vi "Main.vi"() -> ()   [LabVIEW 2018] (continued)
              }
              frame Enabled {
              }
            }
            n1833 = disable-structure shown="启用" {
              disable-tunnel: [w775 w777] -> w747
              disable-tunnel: w743 -> [w774 w777]
              frame Disabled {
                n1834 = call <vilib>:"Boolean Crossing PtByPt.vi"("direction"=enum16{"either", "false-true", "true-false"}."true-false", "input"=w774) -> ("crossing"=w775:bool)  [unwired: 1 in]
              }
              frame Enabled {
              }
            }
            n1835 = call <vilib>:"Boolean Crossing PtByPt.vi"("direction"=enum16{"either", "false-true", "true-false"}."false-true", "input"=w746) -> ("crossing"=w752:bool)  [unwired: 1 in]
            n1836 = case shown="真" w752 {
              tunnel: w754 -> [w815 w820]
              tunnel: w753 -> [w814 w821]
              tunnel: [w815 w819] -> w751
              tunnel: [w814 w818] -> w750
              frame False {
              }
              frame True {
                w829 = u16 0 items=["byte", "word", "Dword"] ("数据类型")
                w827 = u8 132 items=["I/O (P)"=128, "Input (I)"=129, "Output (Q)"=130, "Bit Memory (M)"=131, "Data (DB)"=132, "Instance Data (DI)"=133, "Local Data (L)"=134, "Predecessor Local Data (VL)"=135] ("寄存器类型")
                n1837 = call "S7_Read.vi"("TCP"=w820, "DB #"=u16 20, "读取长度"=u16 13, "寄存器类型"=w827, "起始地址"=u32 6, "数据类型"=w829, "error in"=w821) -> ("TCP"=w819:refnum<k5>, "数据"=w824:u32[], "error out"=w822:errorcluster)  [unwired: 5 in, 1 out]
                n1838 = To Unsigned Word Integer(number=w824) -> (unsigned 16bit integer=w823:u16[])
                n1839 = call "还原为字符串.vi"("error in (no error)"=w822, "输入数组"=w823) -> ("error out"=w817:errorcluster, "字符串"=w816:string)  [unwired: 8 in]
                n1840 = stacked-sequence {
                  tunnel: [_ w833] -> w818
                  tunnel: w817 -> [_ w832]
                  tunnel: w816 -> [w830 _]
                  frame #0 {
                    "80二维码" <- w830
                  }
                  frame #1 {
                    n1841 = property on="ST80扫码请求 （事件）" class="Bool (严格)"(error in=w832, "Val(Sgnl)"=TRUE ("值(信号)")) -> (error out=w833:errorcluster)  [unwired: 1 in, 1 out]
                  }
                }
              }
            }
            n1842 = case shown="假" w744 {
              frame False {
                n1843 = local write "80扫码回复写入"(FALSE ("201扫码回复写入")) -> ()
              }
              frame True {
              }
            }
            n1844 = case shown="假" w747 {
              frame False {
                n1845 = local write "80数据回复写入"(FALSE ("201数据回复写入")) -> ()
              }
              frame True {
              }
            }
            n1846 = call <vilib>:"Boolean Crossing PtByPt.vi"("direction"=enum16{"either", "false-true", "true-false"}."false-true", "input"=w743) -> ("crossing"=w748:bool)  [unwired: 1 in]
            n1847 = case shown="真" w748 {
              tunnel: [w781 w788] -> w742
              tunnel: [w780 w783] -> w741
              tunnel: w750 -> [w780 w789]
              tunnel: w751 -> [w781 w790]
              frame False {
              }
              frame True {
                w794 = u16 1 items=["byte", "word", "Dword"] ("数据类型")
                w796 = u8 132 items=["I/O (P)"=128, "Input (I)"=129, "Output (Q)"=130, "Bit Memory (M)"=131, "Data (DB)"=132, "Instance Data (DI)"=133, "Local Data (L)"=134, "Predecessor Local Data (VL)"=135] ("寄存器类型")
                n1848 = call "S7_Read.vi"("TCP"=w790, "DB #"=u16 20, "读取长度"=u16 1, "寄存器类型"=w796, "起始地址"=u32 20, "数据类型"=w794, "error in"=w789) -> ("TCP"=w788:refnum<k5>, "数据"=w802:u32[], "error out"=w784:errorcluster)  [unwired: 5 in, 1 out]
                n1849 = local read "ST80_Spring_plate_5025473"() -> (w785:string)
                n1850 = local read "ST80_Flat_sael_5020064"() -> (w787:string)
                n1851 = local read "ST80_Spring_5024883"() -> (w786:string)
                n1852 = Index Array(array=w802) -> (element=w804:u32)  [unwired: 1 in]
                n1853 = Equal?(x=w804, y=u32 1) -> (x = y?=w803:bool)
                n1854 = case shown="真" w803 {
                  tunnel: ["NG" "OK"] -> w807
                  frame False {
                  }
                  frame True {
                  }
                }
                n1855 = Format Date/Time String(time format string (%c)="%Y-%m-%d" ("时间格式字符串(%c)")) -> (date/time string=w805:string)  [unwired: 2 in]
                n1856 = Get Date/Time String(want seconds? (F)=TRUE ("需要秒？(F)")) -> (time string=w806:string)  [unwired: 2 in, 1 out]
                n1857 = Insert Into Array(array=string[] [] ("数组"), index=0 ("索引"), new element #1="80" ("新元素/子数组"), new element #2=w807, new element #3=w805, new element #4=w806, new element #5=w807, new element #6=w787, new element #7=w786, new element #8=w785) -> (w782:string[])
                n1858 = stacked-sequence {
                  tunnel: w784 -> [_ w811]
                  tunnel: [_ w810] -> w783
                  tunnel: w782 -> [w808 _]
                  frame #0 {
                    "80数据" <- w808
                  }
                  frame #1 {
                    n1859 = property on="ST80数据保存请求（事件）" class="Bool (严格)"(error in=w811, "Val(Sgnl)"=TRUE ("值(信号)")) -> (error out=w810:errorcluster)  [unwired: 1 in, 1 out]
                  }
                }
              }
            }
          }
          frame "写" {
            w843 = u8 132 items=["I/O (P)"=128, "Input (I)"=129, "Output (Q)"=130, "Bit Memory (M)"=131, "Data (DB)"=132, "Instance Data (DI)"=133, "Local Data (L)"=134, "Predecessor Local Data (VL)"=135] ("寄存器类型")
            w842 = u16 1 items=["byte", "word", "Dword"] ("数据类型")
            w855 = u8 132 items=["I/O (P)"=128, "Input (I)"=129, "Output (Q)"=130, "Bit Memory (M)"=131, "Data (DB)"=132, "Instance Data (DI)"=133, "Local Data (L)"=134, "Predecessor Local Data (VL)"=135] ("寄存器类型")
            w854 = u16 1 items=["byte", "word", "Dword"] ("数据类型")
            w862 = u8 132 items=["I/O (P)"=128, "Input (I)"=129, "Output (Q)"=130, "Bit Memory (M)"=131, "Data (DB)"=132, "Instance Data (DI)"=133, "Local Data (L)"=134, "Predecessor Local Data (VL)"=135] ("寄存器类型")
            w859 = u16 1 items=["byte", "word", "Dword"] ("数据类型")
            n1860 = local read "80看门狗"() -> (w853:i32)
            n1861 = case shown="0" w853 {
              tunnel: [0 ("y") 1 ("y")] -> w852
              frame 1, Default {
              }
              frame 0 {
              }
            }
            "80看门狗" <- w852
            n1862 = call "S7_Write.vi"("TCP"=w858, "寄存器类型"=w862, "DB #"=u16 20, "写入地址"=u32 54, "数据类型"=w859, "写入数据"=w852) -> ("TCP"=w851:refnum<k5>, "error out"=w850:errorcluster)  [unwired: 7 in, 1 out]
            n1863 = case shown="真" "80扫码回复写入" {
              tunnel: w851 -> [w881 w889]
              tunnel: w850 -> [w880 w888]
              tunnel: [w881 w887] -> w848
              tunnel: [w880 w886] -> w847
              tunnel: [999 w885] -> w846
              frame False {
              }
              frame True {
                w897 = u8 132 items=["I/O (P)"=128, "Input (I)"=129, "Output (Q)"=130, "Bit Memory (M)"=131, "Data (DB)"=132, "Instance Data (DI)"=133, "Local Data (L)"=134, "Predecessor Local Data (VL)"=135] ("寄存器类型")
                w896 = u16 1 items=["byte", "word", "Dword"] ("数据类型")
                w891 = u8 132 items=["I/O (P)"=128, "Input (I)"=129, "Output (Q)"=130, "Bit Memory (M)"=131, "Data (DB)"=132, "Instance Data (DI)"=133, "Local Data (L)"=134, "Predecessor Local Data (VL)"=135] ("寄存器类型")
                w892 = u16 1 items=["byte", "word", "Dword"] ("数据类型")
                n1864 = local read "上一站号 (80)"() -> (w884:string)
                n1865 = local read "上一站结果 (80)"() -> (w883:string)
                n1866 = Decimal String To Number(string=w884, default (0L)=u32 0 ("默认(0 I32)")) -> (number=w901:u32)  [unwired: 1 in, 1 out]
                n1867 = call "S7_Write.vi"("TCP"=w889, "寄存器类型"=w891, "DB #"=u16 20, "写入地址"=u32 28, "数据类型"=w892, "写入数据"=w901, "error in"=w888) -> ("TCP"=w900:refnum<k5>, "error out"=w899:errorcluster)  [unwired: 6 in, 1 out]
                n1868 = Equal?(x=w883, y="OK") -> (x = y?=w903:bool)
                n1869 = case shown="假" w903 {
                  tunnel: [u32 2 ("写入数据") u32 1 ("写入数据")] -> w904
                  frame False {
                  }
                  frame True {
                  }
                }
                n1870 = local read "扫码请求回复80"() -> (w882:string)
                n1871 = call "S7_Write.vi"("TCP"=w900, "寄存器类型"=w897, "DB #"=u16 20, "写入地址"=u32 30, "数据类型"=w896, "写入数据"=w904, "error in"=w899) -> ("TCP"=w887:refnum<k5>, "error out"=w886:errorcluster)  [unwired: 6 in, 1 out]
                n1872 = Decimal String To Number(string=w882) -> (number=w885:i32)  [unwired: 2 in, 1 out]
              }
            }
            n1873 = call "S7_Write.vi"("TCP"=w848, "寄存器类型"=w855, "DB #"=u16 20, "写入地址"=u32 2, "数据类型"=w854, "写入数据"=w846, "error in"=w847) -> ("TCP"=w841:refnum<k5>, "error out"=w840:errorcluster)  [unwired: 6 in, 1 out]
            n1874 = case shown="真" "80数据回复写入" {
              tunnel: [999 w878] -> w839
              frame False {
              }
              frame True {
                n1875 = local read "数据保存请求回复80"() -> (w877:string)
                n1876 = Decimal String To Number(string=w877) -> (number=w878:i32)  [unwired: 2 in, 1 out]
              }
            }
            n1877 = call "S7_Write.vi"("TCP"=w841, "寄存器类型"=w843, "DB #"=u16 20, "写入地址"=u32 4, "数据类型"=w842, "写入数据"=w839, "error in"=w840) -> ("TCP"=w837:refnum<k5>, "error out"=w835:errorcluster)  [unwired: 6 in, 1 out]
            n1878 = disable-structure shown="启用" {
              disable-tunnel: w837 -> [w865 w869]
              disable-tunnel: [w865 w872] -> w836
              disable-tunnel: w835 -> [w866 w870]
              disable-tunnel: [w866 w871] -> w834
              frame Disabled {
              }
              frame Enabled {
                w874 = u8 132 items=["I/O (P)"=128, "Input (I)"=129, "Output (Q)"=130, "Bit Memory (M)"=131, "Data (DB)"=132, "Instance Data (DI)"=133, "Local Data (L)"=134, "Predecessor Local Data (VL)"=135] ("寄存器类型")
                w868 = u16 1 items=["byte", "word", "Dword"] ("数据类型")
                n1879 = local read "产品型号"() -> (w867:u32)
                n1880 = call "S7_Write.vi"("TCP"=w869, "寄存器类型"=w874, "DB #"=u16 20, "写入地址"=u32 56, "数据类型"=w868, "写入数据"=w867, "error in"=w870) -> ("TCP"=w872:refnum<k5>, "error out"=w871:errorcluster)  [unwired: 6 in, 1 out]
              }
            }
          }
          frame "错误" {
            n1881 = call "S7_Close.vi"("TCP Connection Ref"=w911) -> ("error out"=w912:errorcluster)  [unwired: 10 in]
            n1882 = call <vilib>:"Clear Errors.vi"("error in (no error)"=w912) -> ()  [unwired: 5 in, 2 out]
          }
          frame "退出" {
            n1883 = call "S7_Close.vi"("TCP Connection Ref"=w918) -> ("error out"=w919:errorcluster)  [unwired: 10 in]
            n1884 = call <vilib>:"Clear Errors.vi"("error in (no error)"=w919) -> ()  [unwired: 5 in, 2 out]
          }
        }
      }
      n1885 = while {
        shift-right: [w2621] -> _
        shift-left: errorcluster {"status"=FALSE, "code"=0, "source"=""} ("错误常量") -> [w2624]
        shift-right: [w2620] -> _
        shift-left: enum16{"初始化", "读", "写", "错误", "退出"}."初始化" -> [w2625]
        shift-right: [w2622] -> _
        shift-left: _ -> [w2619]
        stop <- w2618 stop-if-true
        n1886 = local read "退出"() -> (w2626:bool)
        n1887 = case shown="假" w2626 {
          tunnel: w2625 -> [w2627 _]
          tunnel: [w2628 enum16{"初始化", "读", "写", "错误", "退出"}."退出"] -> w2617
          tunnel: w2624 -> [w2629 _]
          frame False {
            n1888 = case shown="错误" w2629 {
              tunnel: [w2630 enum16{"初始化", "读", "写", "错误", "退出"}."错误"] -> w2628
              tunnel: w2627 -> [w2630 _]
              frame No Error {
              }
              frame Error {
              }
            }
          }
          frame True {
          }
        }
        n1889 = Wait (ms)(milliseconds to wait=u32 80 ("等待时间（毫秒）")) -> ()  [unwired: 1 out]
        n1890 = case shown="\"写\"" w2617 {
          tunnel: [w2635 w2676 w2846 refnum<k5> refnum ("TCP") refnum<k5> refnum ("TCP")] -> w2622
          tunnel: [w2633 w2677 w2844 errorcluster {"status"=FALSE, "code"=0, "source"=""} ("error out") errorcluster {"status"=FALSE, "code"=0, "source"=""} ("error out")] -> w2621
          tunnel: [enum16{"初始化", "读", "写", "错误", "退出"}."读" enum16{"初始化", "读", "写", "错误", "退出"}."写" enum16{"初始化", "读", "写", "错误", "退出"}."读" enum16{"初始化", "读", "写", "错误", "退出"}."初始化" enum16{"初始化", "读", "写", "错误", "退出"}."退出"] -> w2620
          tunnel: w2619 -> [_ w2696 w2886 w2969 w2976]
          tunnel: [FALSE FALSE FALSE FALSE TRUE] -> w2618
          frame "初始化", Default {
            w2648 = u16 0 items=["byte", "word", "Dword"] ("数据类型")
            w2646 = u8 132 items=["I/O (P)"=128, "Input (I)"=129, "Output (Q)"=130, "Bit Memory (M)"=131, "Data (DB)"=132, "Instance Data (DI)"=133, "Local Data (L)"=134, "Predecessor Local Data (VL)"=135] ("寄存器类型")
            w2649 = u16 0 items=["byte", "word", "Dword"] ("数据类型")
            w2651 = u8 132 items=["I/O (P)"=128, "Input (I)"=129, "Output (Q)"=130, "Bit Memory (M)"=131, "Data (DB)"=132, "Instance Data (DI)"=133, "Local Data (L)"=134, "Predecessor Local Data (VL)"=135] ("寄存器类型")
            w2661 = u8 0 items=["S7-1200.200.200SMART"=0, "S7-300"=2, "S7-400"=3] ("PLC 系列")
            n1891 = call "S7_Open.vi"("IP 地址"="192.168.1.40", "PLC 系列"=w2661, "超时（MS）"=100) -> ("TCP"=w2636:refnum<k5>, "error out"=w2634:errorcluster)  [unwired: 10 in, 1 out]
            n1892 = case shown="错误" w2634 {
              tunnel: [FALSE TRUE] -> w2657
              frame No Error {
              }
              frame Error {
              }
            }
            n1893 = local write "ST40通讯状态"(w2657) -> ()
            n1894 = call "S7_Read.vi"("TCP"=w2636, "DB #"=u16 20, "读取长度"=u16 13, "寄存器类型"=w2646, "起始地址"=u32 22, "数据类型"=w2648, "error in"=w2634) -> ("TCP"=w2639:refnum<k5>, "数据"=w2643:u32[], "error out"=w2641:errorcluster)  [unwired: 5 in, 1 out]
            n1895 = To Unsigned Word Integer(number=w2643) -> (unsigned 16bit integer=w2642:u16[])
            n1896 = call "还原为字符串.vi"("error in (no error)"=w2641, "输入数组"=w2642) -> ("error out"=w2638:errorcluster, "字符串"=w2640:string)  [unwired: 8 in]
            n1897 = local write "401二维码"(w2640) -> ()
            n1898 = call "S7_Read.vi"("TCP"=w2639, "DB #"=u16 20, "读取长度"=u16 13, "寄存器类型"=w2651, "起始地址"=u32 44, "数据类型"=w2649, "error in"=w2638) -> ("TCP"=w2635:refnum<k5>, "数据"=w2654:u32[], "error out"=w2656:errorcluster)  [unwired: 5 in, 1 out]
            n1899 = To Unsigned Word Integer(number=w2654) -> (unsigned 16bit integer=w2655:u16[])
            n1900 = call "还原为字符串.vi"("error in (no error)"=w2656, "输入数组"=w2655) -> ("error out"=w2633:errorcluster, "字符串"=w2637:string)  [unwired: 8 in]
            n1901 = local write "402二维码"(w2637) -> ()
          }
          frame "读" {
            w2697 = u16 0 items=["byte", "word", "Dword"] ("数据类型")
            w2699 = u8 132 items=["I/O (P)"=128, "Input (I)"=129, "Output (Q)"=130, "Bit Memory (M)"=131, "Data (DB)"=132, "Instance Data (DI)"=133, "Local Data (L)"=134, "Predecessor Local Data (VL)"=135] ("寄存器类型")
            n1902 = call "S7_Read.vi"("TCP"=w2696, "DB #"=u16 20, "读取长度"=u16 1, "寄存器类型"=w2699, "起始地址"=u32 0, "数据类型"=w2697) -> ("TCP"=w2694:refnum<k5>, "数据"=w2704:u32[], "读取成功"=w2707:bool, "error out"=w2693:errorcluster)  [unwired: 6 in]
            n1903 = Not(x=w2707) -> (.not. x?=→"ST40通讯状态":bool)
            n1904 = Index Array(array=w2704, index=0 ("索引")) -> (element=w2705:u32)
            n1905 = Number To Boolean Array(number=w2705) -> (Boolean array=w2706:bool[])
            n1906 = Index Array(array=w2706, index #1=0 ("索引"), index #5=6 ("索引")) -> (element #1=w2683:bool, element #2=w2671:bool, element #3=w2669:bool, element #4=w2668:bool, element #5=w2666:bool, element #6=w2665:bool)  [unwired: 4 in]
            "ST401扫码请求" <- w2683
            "ST401数据保存请求" <- w2671
            "ST402扫码请求" <- w2669
            "ST402数据保存请求" <- w2668
            n1907 = call <vilib>:"Boolean Crossing PtByPt.vi"("direction"=enum16{"either", "false-true", "true-false"}."false-true", "input"=w2683) -> ("crossing"=w2692:bool)  [unwired: 1 in]
            n1908 = disable-structure shown="启用" {
              disable-tunnel: [w2712 w2713] -> w2684
              disable-tunnel: w2669 -> [w2710 w2713]
              frame Disabled {
                n1909 = call <vilib>:"Boolean Crossing PtByPt.vi"("direction"=enum16{"either", "false-true", "true-false"}."true-false", "input"=w2710) -> ("crossing"=w2712:bool)  [unwired: 1 in]
              }
              frame Enabled {
              }
            }
            n1910 = disable-structure shown="启用" {
              disable-tunnel: [w2723 w2725] -> w2685
              disable-tunnel: w2671 -> [w2722 w2725]
              frame Disabled {
                n1911 = call <vilib>:"Boolean Crossing PtByPt.vi"("direction"=enum16{"either", "false-true", "true-false"}."true-false", "input"=w2722) -> ("crossing"=w2723:bool)  [unwired: 1 in]
              }
              frame Enabled {
              }
            }
            n1912 = case shown="真" w2692 {
              tunnel: w2694 -> [w2825 w2830]
              tunnel: w2693 -> [w2824 w2831]
              tunnel: [w2825 w2829] -> w2691
              tunnel: [w2824 w2828] -> w2690
              frame False {
              }
              frame True {
                w2839 = u16 0 items=["byte", "word", "Dword"] ("数据类型")
                w2837 = u8 132 items=["I/O (P)"=128, "Input (I)"=129, "Output (Q)"=130, "Bit Memory (M)"=131, "Data (DB)"=132, "Instance Data (DI)"=133, "Local Data (L)"=134, "Predecessor Local Data (VL)"=135] ("寄存器类型")
                n1913 = call "S7_Read.vi"("TCP"=w2830, "DB #"=u16 20, "读取长度"=u16 13, "寄存器类型"=w2837, "起始地址"=u32 22, "数据类型"=w2839, "error in"=w2831) -> ("TCP"=w2829:refnum<k5>, "数据"=w2834:u32[], "error out"=w2832:errorcluster)  [unwired: 5 in, 1 out]
                n1914 = To Unsigned Word Integer(number=w2834) -> (unsigned 16bit integer=w2833:u16[])
                n1915 = call "还原为字符串.vi"("error in (no error)"=w2832, "输入数组"=w2833) -> ("error out"=w2827:errorcluster, "字符串"=w2826:string)  [unwired: 8 in]
                n1916 = stacked-sequence {
                  tunnel: [_ w2843] -> w2828
                  tunnel: w2827 -> [_ w2842]
                  tunnel: w2826 -> [w2840 _]
                  frame #0 {
                    "401二维码" <- w2840
                  }
                  frame #1 {
                    n1917 = property on="ST401扫码请求（事件）" class="Bool (严格)"(error in=w2842, "Val(Sgnl)"=TRUE ("值(信号)")) -> (error out=w2843:errorcluster)  [unwired: 1 in, 1 out]
                  }
                }
              }
            }
            n1918 = disable-structure shown="启用" {
              disable-tunnel: enum16{"either", "false-true", "true-false"}."true-false" ("direction") -> [w2716 _]
              disable-tunnel: w2683 -> [w2715 w2717]
              disable-tunnel: [w2714 w2717] -> w2672
              frame Disabled {
                n1919 = call <vilib>:"Boolean Crossing PtByPt.vi"("direction"=w2716, "input"=w2715) -> ("crossing"=w2714:bool)  [unwired: 1 in]
              }
              frame Enabled {
              }
            }
            n1920 = case shown="假" w2672 {
              frame False {
                n1921 = local write "401扫码回复写入"(FALSE ("201扫码回复写入")) -> ()
              }
              frame True {
              }
            }
            n1922 = case shown="假" w2684 {
              frame False {
                n1923 = local write "402扫码回复写入"(FALSE ("202扫码回复写入")) -> ()
              }
              frame True {
              }
            }
            n1924 = case shown="假" w2685 {
              frame False {
                n1925 = local write "401数据回复写入"(FALSE ("201数据回复写入")) -> ()
              }
              frame True {
              }
            }
            n1926 = disable-structure shown="启用" {
              disable-tunnel: [w2719 w2721] -> w2670
              disable-tunnel: w2668 -> [w2718 w2721]
              frame Disabled {
                n1927 = call <vilib>:"Boolean Crossing PtByPt.vi"("direction"=enum16{"either", "false-true", "true-false"}."true-false", "input"=w2718) -> ("crossing"=w2719:bool)  [unwired: 1 in]
              }
              frame Enabled {
              }
            }
            n1928 = call <vilib>:"Boolean Crossing PtByPt.vi"("direction"=enum16{"either", "false-true", "true-false"}."false-true", "input"=w2671) -> ("crossing"=w2688:bool)  [unwired: 1 in]
            n1929 = case shown="真" w2688 {
              tunnel: [w2788 w2796] -> w2682
              tunnel: [w2787 w2790] -> w2681
              tunnel: w2690 -> [w2787 w2797]
              tunnel: w2691 -> [w2788 w2798]
              tunnel: w2666 -> [_ w2793]
              frame False {
              }
              frame True {
                w2802 = u16 1 items=["byte", "word", "Dword"] ("数据类型")
                w2804 = u8 132 items=["I/O (P)"=128, "Input (I)"=129, "Output (Q)"=130, "Bit Memory (M)"=131, "Data (DB)"=132, "Instance Data (DI)"=133, "Local Data (L)"=134, "Predecessor Local Data (VL)"=135] ("寄存器类型")
                n1930 = case shown="假" w2793 {
                  tunnel: ["F" "T"] -> w2792
                  frame False {
                  }
                  frame True {
                  }
                }
                n1931 = call "S7_Read.vi"("TCP"=w2798, "DB #"=u16 20, "读取长度"=u16 2, "寄存器类型"=w2804, "起始地址"=u32 64, "数据类型"=w2802, "error in"=w2797) -> ("TCP"=w2796:refnum<k5>, "数据"=w2810:u32[], "error out"=w2791:errorcluster)  [unwired: 5 in, 1 out]
                n1932 = Index Array(array=w2810) -> (element #1=w2812:u32, element #2=w2795:u32)  [unwired: 2 in]
                n1933 = Equal?(x=w2812, y=u32 1) -> (x = y?=w2811:bool)
                n1934 = case shown="真" w2811 {
                  tunnel: ["NG" "OK"] -> w2815
                  frame False {
                  }
                  frame True {
                  }
                }
                n1935 = Number To Decimal String(number=w2795) -> (decimal integer string=w2794:string)  [unwired: 1 in]
                n1936 = Format Date/Time String(time format string (%c)="%Y-%m-%d" ("时间格式字符串(%c)")) -> (date/time string=w2813:string)  [unwired: 2 in]
                n1937 = Get Date/Time String(want seconds? (F)=TRUE ("需要秒？(F)")) -> (time string=w2814:string)  [unwired: 2 in, 1 out]
                n1938 = Insert Into Array(array=string[] [] ("数组"), index=0 ("索引"), new element #1="401" ("新元素/子数组"), new element #2=w2815, new element #3=w2813, new element #4=w2814, new element #5=w2815, new element #6=w2794, new element #7=w2792) -> (w2789:string[])
                n1939 = stacked-sequence {
                  tunnel: w2791 -> [_ w2819]
                  tunnel: [_ w2818] -> w2790
                  tunnel: w2789 -> [w2816 _]
                  frame #0 {
                    "401数据" <- w2816
                  }
                  frame #1 {
                    n1940 = property on="ST401数据读取（事件）" class="Bool (严格)"(error in=w2819, "Val(Sgnl)"=TRUE ("值(信号)")) -> (error out=w2818:errorcluster)  [unwired: 1 in, 1 out]
                  }
                }
              }
            }
            n1941 = case shown="假" w2670 {
              frame False {
                n1942 = local write "402数据回复写入"(FALSE ("202数据回复写入")) -> ()
              }
              frame True {
              }
            }
            n1943 = call <vilib>:"Boolean Crossing PtByPt.vi"("direction"=enum16{"either", "false-true", "true-false"}."false-true", "input"=w2669) -> ("crossing"=w2680:bool)  [unwired: 1 in]
            n1944 = case shown="真" w2680 {
              tunnel: w2682 -> [w2765 w2771]
              tunnel: w2681 -> [w2764 w2770]
              tunnel: [w2764 w2767] -> w2678
              tunnel: [w2765 w2769] -> w2679
              frame False {
              }
              frame True {
                w2772 = u16 0 items=["byte", "word", "Dword"] ("数据类型")
                w2774 = u8 132 items=["I/O (P)"=128, "Input (I)"=129, "Output (Q)"=130, "Bit Memory (M)"=131, "Data (DB)"=132, "Instance Data (DI)"=133, "Local Data (L)"=134, "Predecessor Local Data (VL)"=135] ("寄存器类型")
                n1945 = call "S7_Read.vi"("TCP"=w2771, "DB #"=u16 20, "读取长度"=u16 13, "寄存器类型"=w2774, "起始地址"=u32 44, "数据类型"=w2772, "error in"=w2770) -> ("TCP"=w2769:refnum<k5>, "数据"=w2777:u32[], "error out"=w2779:errorcluster)  [unwired: 5 in, 1 out]
                n1946 = To Unsigned Word Integer(number=w2777) -> (unsigned 16bit integer=w2778:u16[])
                n1947 = call "还原为字符串.vi"("error in (no error)"=w2779, "输入数组"=w2778) -> ("error out"=w2768:errorcluster, "字符串"=w2766:string)  [unwired: 8 in]
                n1948 = stacked-sequence {
                  tunnel: w2768 -> [_ w2783]
                  tunnel: [_ w2781] -> w2767
                  tunnel: w2766 -> [w2780 _]
                  frame #0 {
                    "402二维码" <- w2780
                  }
                  frame #1 {
                    n1949 = property on="ST402扫码请求（事件）" class="Bool (严格)"(error in=w2783, "Val(Sgnl)"=TRUE ("值(信号)")) -> (error out=w2781:errorcluster)  [unwired: 1 in, 1 out]
                  }
                }
              }
            }
            n1950 = call <vilib>:"Boolean Crossing PtByPt.vi"("direction"=enum16{"either", "false-true", "true-false"}."false-true", "input"=w2668) -> ("crossing"=w2674:bool)  [unwired: 1 in]
            n1951 = case shown="真" w2674 {
              tunnel: w2679 -> [w2728 w2735]
              tunnel: w2678 -> [w2727 w2734]
              tunnel: [w2728 w2733] -> w2676
              tunnel: [w2727 w2730] -> w2677
              tunnel: w2665 -> [_ w2732]
              frame False {
              }
              frame True {
                w2749 = u16 1 items=["byte", "word", "Dword"] ("数据类型")
                w2747 = u8 132 items=["I/O (P)"=128, "Input (I)"=129, "Output (Q)"=130, "Bit Memory (M)"=131, "Data (DB)"=132, "Instance Data (DI)"=133, "Local Data (L)"=134, "Predecessor Local Data (VL)"=135] ("寄存器类型")
                n1952 = call "S7_Read.vi"("TCP"=w2735, "DB #"=u16 20, "读取长度"=u16 2, "寄存器类型"=w2747, "起始地址"=u32 68, "数据类型"=w2749, "error in"=w2734) -> ("TCP"=w2733:refnum<k5>, "数据"=w2741:u32[], "error out"=w2731:errorcluster)  [unwired: 5 in, 1 out]
                n1953 = case shown="假" w2732 {
                  tunnel: ["F" "T"] -> w2755
                  frame False {
                  }
                  frame True {
                  }
                }
                n1954 = Index Array(array=w2741) -> (element #1=w2739:u32, element #2=w2753:u32)  [unwired: 2 in]
                n1955 = Equal?(x=w2739, y=u32 1) -> (x = y?=w2740:bool)
                n1956 = case shown="真" w2740 {
                  tunnel: ["NG" "OK"] -> w2736
                  frame False {
                  }
                  frame True {
                  }
                }
                n1957 = Number To Decimal String(number=w2753) -> (decimal integer string=w2754:string)  [unwired: 1 in]
                n1958 = Format Date/Time String(time format string (%c)="%Y-%m-%d" ("时间格式字符串(%c)")) -> (date/time string=w2738:string)  [unwired: 2 in]
                n1959 = Get Date/Time String(want seconds? (F)=TRUE ("需要秒？(F)")) -> (time string=w2737:string)  [unwired: 2 in, 1 out]
                n1960 = Insert Into Array(array=string[] [] ("数组"), index=0 ("索引"), new element #1="402" ("新元素/子数组"), new element #2=w2736, new element #3=w2738, new element #4=w2737, new element #5=w2736, new element #6=w2754, new element #7=w2755) -> (w2729:string[])
                n1961 = stacked-sequence {
                  tunnel: w2731 -> [_ w2759]
                  tunnel: [_ w2758] -> w2730
                  tunnel: w2729 -> [w2756 _]
                  frame #0 {
                    "402data" <- w2756
                  }
                  frame #1 {
                    n1962 = property on="ST402数据读取（事件）" class="Bool (严格)"(error in=w2759, "Val(Sgnl)"=TRUE ("值(信号)")) -> (error out=w2758:errorcluster)  [unwired: 1 in, 1 out]
                  }
                }
              }
            }
          }
          frame "写" {
            w2855 = u8 132 items=["I/O (P)"=128, "Input (I)"=129, "Output (Q)"=130, "Bit Memory (M)"=131, "Data (DB)"=132, "Instance Data (DI)"=133, "Local Data (L)"=134, "Predecessor Local Data (VL)"=135] ("寄存器类型")
            w2854 = u16 1 items=["byte", "word", "Dword"] ("数据类型")
            w2872 = u8 132 items=["I/O (P)"=128, "Input (I)"=129, "Output (Q)"=130, "Bit Memory (M)"=131, "Data (DB)"=132, "Instance Data (DI)"=133, "Local Data (L)"=134, "Predecessor Local Data (VL)"=135] ("寄存器类型")
            w2873 = u16 1 items=["byte", "word", "Dword"] ("数据类型")
            w2880 = u8 132 items=["I/O (P)"=128, "Input (I)"=129, "Output (Q)"=130, "Bit Memory (M)"=131, "Data (DB)"=132, "Instance Data (DI)"=133, "Local Data (L)"=134, "Predecessor Local Data (VL)"=135] ("寄存器类型")
            w2881 = u16 1 items=["byte", "word", "Dword"] ("数据类型")
            w2883 = u8 132 items=["I/O (P)"=128, "Input (I)"=129, "Output (Q)"=130, "Bit Memory (M)"=131, "Data (DB)"=132, "Instance Data (DI)"=133, "Local Data (L)"=134, "Predecessor Local Data (VL)"=135] ("寄存器类型")
            w2882 = u16 1 items=["byte", "word", "Dword"] ("数据类型")
            w2890 = u8 132 items=["I/O (P)"=128, "Input (I)"=129, "Output (Q)"=130, "Bit Memory (M)"=131, "Data (DB)"=132, "Instance Data (DI)"=133, "Local Data (L)"=134, "Predecessor Local Data (VL)"=135] ("寄存器类型")
            w2887 = u16 1 items=["byte", "word", "Dword"] ("数据类型")
            n1963 = local read "40看门狗"() -> (w2865:i32)
            n1964 = case shown="0" w2865 {
              tunnel: [0 ("y") 1 ("y")] -> w2864
              frame 1, Default {
              }
              frame 0 {
              }
            }
            "40看门狗" <- w2864
            n1965 = call "S7_Write.vi"("TCP"=w2886, "寄存器类型"=w2890, "DB #"=u16 20, "写入地址"=u32 2, "数据类型"=w2887, "写入数据"=w2864) -> ("TCP"=w2863:refnum<k5>, "error out"=w2862:errorcluster)  [unwired: 7 in, 1 out]
            n1966 = case shown="真" "401扫码回复写入" {
              tunnel: w2863 -> [w2909 w2917]
              tunnel: w2862 -> [w2908 w2916]
              tunnel: [w2909 w2915] -> w2860
              tunnel: [w2908 w2914] -> w2859
              tunnel: [999 w2913] -> w2858
              frame False {
              }
              frame True {
                w2925 = u8 132 items=["I/O (P)"=128, "Input (I)"=129, "Output (Q)"=130, "Bit Memory (M)"=131, "Data (DB)"=132, "Instance Data (DI)"=133, "Local Data (L)"=134, "Predecessor Local Data (VL)"=135] ("寄存器类型")
                w2924 = u16 1 items=["byte", "word", "Dword"] ("数据类型")
                w2919 = u8 132 items=["I/O (P)"=128, "Input (I)"=129, "Output (Q)"=130, "Bit Memory (M)"=131, "Data (DB)"=132, "Instance Data (DI)"=133, "Local Data (L)"=134, "Predecessor Local Data (VL)"=135] ("寄存器类型")
                w2920 = u16 1 items=["byte", "word", "Dword"] ("数据类型")
                n1967 = local read "上一站号 (401)"() -> (w2912:string)
                n1968 = local read "上一站结果 (401)"() -> (w2911:string)
                n1969 = Decimal String To Number(string=w2912, default (0L)=u32 0 ("默认(0 I32)")) -> (number=w2929:u32)  [unwired: 1 in, 1 out]
                n1970 = call "S7_Write.vi"("TCP"=w2917, "寄存器类型"=w2919, "DB #"=u16 20, "写入地址"=u32 12, "数据类型"=w2920, "写入数据"=w2929, "error in"=w2916) -> ("TCP"=w2928:refnum<k5>, "error out"=w2927:errorcluster)  [unwired: 6 in, 1 out]
                n1971 = Equal?(x=w2911, y="OK") -> (x = y?=w2931:bool)
                n1972 = case shown="假" w2931 {
                  tunnel: [u32 2 ("写入数据") u32 1 ("写入数据")] -> w2932
                  frame False {
                  }
                  frame True {
                  }
                }
                n1973 = local read "扫码请求回复401"() -> (w2910:string)
                n1974 = call "S7_Write.vi"("TCP"=w2928, "寄存器类型"=w2925, "DB #"=u16 20, "写入地址"=u32 14, "数据类型"=w2924, "写入数据"=w2932, "error in"=w2927) -> ("TCP"=w2915:refnum<k5>, "error out"=w2914:errorcluster)  [unwired: 6 in, 1 out]
                n1975 = Decimal String To Number(string=w2910) -> (number=w2913:i32)  [unwired: 2 in, 1 out]
              }
            }
            n1976 = call "S7_Write.vi"("TCP"=w2860, "寄存器类型"=w2883, "DB #"=u16 20, "写入地址"=u32 4, "数据类型"=w2882, "写入数据"=w2858, "error in"=w2859) -> ("TCP"=w2853:refnum<k5>, "error out"=w2852:errorcluster)  [unwired: 6 in, 1 out]
            n1977 = case shown="真" "401数据回复写入" {
              tunnel: [999 w2906] -> w2851
              frame False {
              }
              frame True {
                n1978 = local read "数据保存请求回复401"() -> (w2905:string)
                n1979 = Decimal String To Number(string=w2905) -> (number=w2906:i32)  [unwired: 2 in, 1 out]
              }
            }
            n1980 = call "S7_Write.vi"("TCP"=w2853, "寄存器类型"=w2855, "DB #"=u16 20, "写入地址"=u32 6, "数据类型"=w2854, "写入数据"=w2851, "error in"=w2852) -> ("TCP"=w2849:refnum<k5>, "error out"=w2848:errorcluster)  [unwired: 6 in, 1 out]
            n1981 = case shown="真" "402扫码回复写入" {
              tunnel: [999 w2944] -> w2876
              tunnel: w2849 -> [w2939 w2958]
              tunnel: w2848 -> [w2938 w2957]
              tunnel: [w2939 w2946] -> w2875
              tunnel: [w2938 w2945] -> w2874
              frame False {
              }
              frame True {
                w2952 = u8 132 items=["I/O (P)"=128, "Input (I)"=129, "Output (Q)"=130, "Bit Memory (M)"=131, "Data (DB)"=132, "Instance Data (DI)"=133, "Local Data (L)"=134, "Predecessor Local Data (VL)"=135] ("寄存器类型")
                w2953 = u16 1 items=["byte", "word", "Dword"] ("数据类型")
                w2960 = u8 132 items=["I/O (P)"=128, "Input (I)"=129, "Output (Q)"=130, "Bit Memory (M)"=131, "Data (DB)"=132, "Instance Data (DI)"=133, "Local Data (L)"=134, "Predecessor Local Data (VL)"=135] ("寄存器类型")
                w2959 = u16 1 items=["byte", "word", "Dword"] ("数据类型")
                n1982 = local read "上一站号 (402)"() -> (w2943:string)
                n1983 = Decimal String To Number(string=w2943) -> (number=w2956:i32)  [unwired: 2 in, 1 out]
                n1984 = call "S7_Write.vi"("TCP"=w2958, "寄存器类型"=w2960, "DB #"=u16 20, "写入地址"=u32 16, "数据类型"=w2959, "写入数据"=w2956, "error in"=w2957) -> ("TCP"=w2948:refnum<k5>, "error out"=w2949:errorcluster)  [unwired: 6 in, 1 out]
                n1985 = local read "上一站结果 (402)"() -> (w2942:string)
                n1986 = local read "扫码请求回复402"() -> (w2941:string)
                n1987 = Equal?(x=w2942, y="OK") -> (x = y?=w2955:bool)
                n1988 = case shown="假" w2955 {
                  tunnel: [u32 2 ("写入数据") u32 1 ("写入数据")] -> w2947
                  frame False {
                  }
                  frame True {
                  }
                }
                n1989 = call "S7_Write.vi"("TCP"=w2948, "寄存器类型"=w2952, "DB #"=u16 20, "写入地址"=u32 18, "数据类型"=w2953, "写入数据"=w2947, "error in"=w2949) -> ("TCP"=w2946:refnum<k5>, "error out"=w2945:errorcluster)  [unwired: 6 in, 1 out]
                n1990 = Decimal String To Number(string=w2941) -> (number=w2944:i32)  [unwired: 2 in, 1 out]
              }
            }
            n1991 = call "S7_Write.vi"("TCP"=w2875, "寄存器类型"=w2880, "DB #"=u16 20, "写入地址"=u32 8, "数据类型"=w2881, "写入数据"=w2876, "error in"=w2874) -> ("TCP"=w2868:refnum<k5>, "error out"=w2869:errorcluster)  [unwired: 6 in, 1 out]
            n1992 = case shown="真" "402数据回复写入" {
              tunnel: [999 w2937] -> w2866
              frame False {
              }
              frame True {
                n1993 = local read "数据保存请求回复402"() -> (w2936:string)
                n1994 = Decimal String To Number(string=w2936) -> (number=w2937:i32)  [unwired: 2 in, 1 out]
              }
            }
            n1995 = call "S7_Write.vi"("TCP"=w2868, "寄存器类型"=w2872, "DB #"=u16 20, "写入地址"=u32 10, "数据类型"=w2873, "写入数据"=w2866, "error in"=w2869) -> ("TCP"=w2847:refnum<k5>, "error out"=w2845:errorcluster)  [unwired: 6 in, 1 out]
            n1996 = disable-structure shown="启用" {
              disable-tunnel: w2847 -> [w2893 w2897]
              disable-tunnel: [w2893 w2900] -> w2846
              disable-tunnel: w2845 -> [w2894 w2898]
              disable-tunnel: [w2894 w2899] -> w2844
              frame Disabled {
              }
              frame Enabled {
                w2902 = u8 132 items=["I/O (P)"=128, "Input (I)"=129, "Output (Q)"=130, "Bit Memory (M)"=131, "Data (DB)"=132, "Instance Data (DI)"=133, "Local Data (L)"=134, "Predecessor Local Data (VL)"=135] ("寄存器类型")
                w2896 = u16 1 items=["byte", "word", "Dword"] ("数据类型")
                n1997 = local read "产品型号"() -> (w2895:u32)
                n1998 = call "S7_Write.vi"("TCP"=w2897, "寄存器类型"=w2902, "DB #"=u16 20, "写入地址"=u32 72, "数据类型"=w2896, "写入数据"=w2895, "error in"=w2898) -> ("TCP"=w2900:refnum<k5>, "error out"=w2899:errorcluster)  [unwired: 6 in, 1 out]
              }
            }
          }
          frame "错误" {
            n1999 = call "S7_Close.vi"("TCP Connection Ref"=w2969) -> ("error out"=w2970:errorcluster)  [unwired: 10 in]
            n2000 = call <vilib>:"Clear Errors.vi"("error in (no error)"=w2970) -> ()  [unwired: 5 in, 2 out]
          }
          frame "退出" {
            n2001 = call "S7_Close.vi"("TCP Connection Ref"=w2976) -> ("error out"=w2977:errorcluster)  [unwired: 10 in]
            n2002 = call <vilib>:"Clear Errors.vi"("error in (no error)"=w2977) -> ()  [unwired: 5 in, 2 out]
          }
        }
      }
      n2003 = while {
        shift-right: [w3543] -> _
        shift-left: errorcluster {"status"=FALSE, "code"=0, "source"=""} ("错误常量") -> [w3546]
        shift-right: [w3542] -> _
        shift-left: enum16{"初始化", "读", "写", "错误", "退出"}."初始化" -> [w3547]
        shift-right: [w3544] -> _
        shift-left: _ -> [w3541]
        stop <- w3540 stop-if-true
        n2004 = local read "退出"() -> (w3548:bool)
        n2005 = case shown="假" w3548 {
          tunnel: w3547 -> [w3549 _]
          tunnel: [w3550 enum16{"初始化", "读", "写", "错误", "退出"}."退出"] -> w3539
          tunnel: w3546 -> [w3551 _]
          frame False {
            n2006 = case shown="错误" w3551 {
              tunnel: [w3552 enum16{"初始化", "读", "写", "错误", "退出"}."错误"] -> w3550
              tunnel: w3549 -> [w3552 _]
              frame No Error {
              }
              frame Error {
              }
            }
          }
          frame True {
          }
        }
        n2007 = Wait (ms)(milliseconds to wait=u32 80 ("等待时间（毫秒）")) -> ()  [unwired: 1 out]
        n2008 = case shown="\"写\"" w3539 {
          tunnel: [w3555 w3594 w3904 refnum<k5> refnum ("TCP") refnum<k5> refnum ("TCP")] -> w3544
          tunnel: [w3556 w3595 w3902 errorcluster {"status"=FALSE, "code"=0, "source"=""} ("error out") errorcluster {"status"=FALSE, "code"=0, "source"=""} ("error out")] -> w3543
          tunnel: [enum16{"初始化", "读", "写", "错误", "退出"}."读" enum16{"初始化", "读", "写", "错误", "退出"}."写" enum16{"初始化", "读", "写", "错误", "退出"}."读" enum16{"初始化", "读", "写", "错误", "退出"}."初始化" enum16{"初始化", "读", "写", "错误", "退出"}."退出"] -> w3542
          tunnel: w3541 -> [_ w3613 w3906 w4036 w4043]
          tunnel: [FALSE FALSE FALSE FALSE TRUE] -> w3540
          frame "初始化", Default {
            w3569 = u16 0 items=["byte", "word", "Dword"] ("数据类型")
            w3567 = u8 132 items=["I/O (P)"=128, "Input (I)"=129, "Output (Q)"=130, "Bit Memory (M)"=131, "Data (DB)"=132, "Instance Data (DI)"=133, "Local Data (L)"=134, "Predecessor Local Data (VL)"=135] ("寄存器类型")
            w3577 = u16 0 items=["byte", "word", "Dword"] ("数据类型")
            w3575 = u8 132 items=["I/O (P)"=128, "Input (I)"=129, "Output (Q)"=130, "Bit Memory (M)"=131, "Data (DB)"=132, "Instance Data (DI)"=133, "Local Data (L)"=134, "Predecessor Local Data (VL)"=135] ("寄存器类型")
            w3583 = u8 0 items=["S7-1200.200.200SMART"=0, "S7-300"=2, "S7-400"=3] ("PLC 系列")
            n2009 = call "S7_Open.vi"("IP 地址"="192.168.1.20", "PLC 系列"=w3583, "超时（MS）"=100) -> ("TCP"=w3560:refnum<k5>, "error out"=w3559:errorcluster)  [unwired: 10 in, 1 out]
            n2010 = call "S7_Read.vi"("TCP"=w3560, "DB #"=u16 20, "读取长度"=u16 13, "寄存器类型"=w3575, "起始地址"=u32 22, "数据类型"=w3577, "error in"=w3559) -> ("TCP"=w3558:refnum<k5>, "数据"=w3572:u32[], "error out"=w3570:errorcluster)  [unwired: 5 in, 1 out]
            n2011 = To Unsigned Word Integer(number=w3572) -> (unsigned 16bit integer=w3571:u16[])
            n2012 = call "还原为字符串.vi"("error in (no error)"=w3570, "输入数组"=w3571) -> ("error out"=w3557:errorcluster, "字符串"=w3578:string)  [unwired: 8 in]
            n2013 = local write "201二维码"(w3578) -> ()
            n2014 = call "S7_Read.vi"("TCP"=w3558, "DB #"=u16 20, "读取长度"=u16 13, "寄存器类型"=w3567, "起始地址"=u32 44, "数据类型"=w3569, "error in"=w3557) -> ("TCP"=w3555:refnum<k5>, "数据"=w3564:u32[], "error out"=w3562:errorcluster)  [unwired: 5 in, 1 out]
            n2015 = To Unsigned Word Integer(number=w3564) -> (unsigned 16bit integer=w3563:u16[])
            n2016 = call "还原为字符串.vi"("error in (no error)"=w3562, "输入数组"=w3563) -> ("error out"=w3556:errorcluster, "字符串"=w3561:string)  [unwired: 8 in]
            n2017 = local write "202二维码"(w3561) -> ()
            n2018 = case shown="错误" w3556 {
              tunnel: [FALSE TRUE] -> w3579
              frame No Error {
              }
              frame Error {
              }
            }
            n2019 = local write "ST20通讯状态"(w3579) -> ()
          }
          frame "读" {
            w3614 = u16 0 items=["byte", "word", "Dword"] ("数据类型")
            w3616 = u8 132 items=["I/O (P)"=128, "Input (I)"=129, "Output (Q)"=130, "Bit Memory (M)"=131, "Data (DB)"=132, "Instance Data (DI)"=133, "Local Data (L)"=134, "Predecessor Local Data (VL)"=135] ("寄存器类型")
            n2020 = call "S7_Read.vi"("TCP"=w3613, "DB #"=u16 20, "读取长度"=u16 1, "寄存器类型"=w3616, "起始地址"=u32 0, "数据类型"=w3614) -> ("TCP"=w3611:refnum<k5>, "数据"=w3621:u32[], "读取成功"=w3624:bool, "error out"=w3610:errorcluster)  [unwired: 6 in]
            n2021 = Not(x=w3624) -> (.not. x?=→"ST20通讯状态":bool)
            n2022 = Index Array(array=w3621, index=0 ("索引")) -> (element=w3622:u32)
            n2023 = Number To Boolean Array(number=w3622) -> (Boolean array=w3623:bool[])
            n2024 = Index Array(array=w3623, index #1=0 ("索引")) -> (element #1=w3601:bool, element #2=w3589:bool, element #3=w3588:bool, element #4=w3587:bool)  [unwired: 3 in]
            "ST201扫码请求" <- w3601
            "ST201数据保存请求" <- w3589
            "ST202扫码请求" <- w3588
            "ST202数据保存请求" <- w3587
            n2025 = disable-structure shown="启用" {
              disable-tunnel: w3601 -> [w3632 w3634]
              disable-tunnel: [w3631 w3634] -> w3590
              frame Disabled {
                n2026 = call <vilib>:"Boolean Crossing PtByPt.vi"("direction"=enum16{"either", "false-true", "true-false"}."true-false", "input"=w3632) -> ("crossing"=w3631:bool)  [unwired: 1 in]
              }
              frame Enabled {
              }
            }
            n2027 = disable-structure shown="禁用" {
              disable-tunnel: [w3636 w3638] -> w3603
              disable-tunnel: w3589 -> [w3635 w3638]
              frame Disabled {
                n2028 = call <vilib>:"Boolean Crossing PtByPt.vi"("direction"=enum16{"either", "false-true", "true-false"}."true-false", "input"=w3635) -> ("crossing"=w3636:bool)  [unwired: 1 in]
              }
              frame Enabled {
              }
            }
            n2029 = call <vilib>:"Boolean Crossing PtByPt.vi"("direction"=enum16{"either", "false-true", "true-false"}."false-true", "input"=w3601) -> ("crossing"=w3609:bool)  [unwired: 1 in]
            n2030 = disable-structure shown="启用" {
              disable-tunnel: [w3629 w3630] -> w3602
              disable-tunnel: w3588 -> [w3627 w3630]
              frame Disabled {
                n2031 = call <vilib>:"Boolean Crossing PtByPt.vi"("direction"=enum16{"either", "false-true", "true-false"}."true-false", "input"=w3627) -> ("crossing"=w3629:bool)  [unwired: 1 in]
              }
              frame Enabled {
              }
            }
            n2032 = case shown="真" w3609 {
              tunnel: w3611 -> [w3881 w3886]
              tunnel: w3610 -> [w3880 w3887]
              tunnel: [w3881 w3884] -> w3608
              tunnel: [w3880 w3883] -> w3607
              frame False {
              }
              frame True {
                w3895 = u16 0 items=["byte", "word", "Dword"] ("数据类型")
                w3893 = u8 132 items=["I/O (P)"=128, "Input (I)"=129, "Output (Q)"=130, "Bit Memory (M)"=131, "Data (DB)"=132, "Instance Data (DI)"=133, "Local Data (L)"=134, "Predecessor Local Data (VL)"=135] ("寄存器类型")
                n2033 = call "S7_Read.vi"("TCP"=w3886, "DB #"=u16 20, "读取长度"=u16 13, "寄存器类型"=w3893, "起始地址"=u32 22, "数据类型"=w3895, "error in"=w3887) -> ("TCP"=w3884:refnum<k5>, "数据"=w3890:u32[], "error out"=w3888:errorcluster)  [unwired: 5 in, 1 out]
                n2034 = To Unsigned Word Integer(number=w3890) -> (unsigned 16bit integer=w3889:u16[])
                n2035 = call "还原为字符串.vi"("error in (no error)"=w3888, "输入数组"=w3889) -> ("error out"=w3885:errorcluster, "字符串"=w3882:string)  [unwired: 8 in]
                n2036 = stacked-sequence {
                  tunnel: w3885 -> [_ w3898]
                  tunnel: [_ w3897] -> w3883
                  tunnel: w3882 -> [w3896 _]
                  frame #0 {
                    "201二维码" <- w3896
                  }
                  frame #1 {
                    n2037 = property on="ST201扫码请求(事件)" class="Bool (严格)"(error in=w3898, "Val(Sgnl)"=TRUE ("值(信号)")) -> (error out=w3897:errorcluster)  [unwired: 1 in, 1 out]
                  }
                }
              }
            }
            n2038 = case shown="假" w3590 {
              frame False {
                n2039 = local write "201扫码回复写入"(FALSE ("201扫码回复写入")) -> ()
              }
              frame True {
              }
            }
            n2040 = case shown="假" w3602 {
              frame False {
                n2041 = local write "202扫码回复写入"(FALSE ("202扫码回复写入")) -> ()
              }
              frame True {
              }
            }
            n2042 = case shown="假" w3603 {
              frame False {
                n2043 = local write "201数据回复写入"(FALSE ("201数据回复写入")) -> ()
              }
              frame True {
              }
            }
            n2044 = disable-structure shown="启用" {
              disable-tunnel: w3587 -> [w3639 w3643]
              frame Disabled {
                n2045 = call <vilib>:"Boolean Crossing PtByPt.vi"("direction"=enum16{"either", "false-true", "true-false"}."true-false", "input"=w3639) -> ("crossing"=w3640:bool)  [unwired: 1 in]
                n2046 = case shown="真" w3640 {
                  frame False {
                  }
                  frame True {
                    n2047 = local write "202数据回复写入"(FALSE ("202数据回复写入")) -> ()
                  }
                }
              }
              frame Enabled {
                n2048 = case shown="假" w3643 {
                  frame False {
                    n2049 = local write "202数据回复写入"(FALSE ("202数据回复写入")) -> ()
                  }
                  frame True {
                  }
                }
              }
            }
            n2050 = call <vilib>:"Boolean Crossing PtByPt.vi"("direction"=enum16{"either", "false-true", "true-false"}."false-true", "input"=w3589) -> ("crossing"=w3605:bool)  [unwired: 1 in]
            n2051 = case shown="真" w3605 {
              tunnel: [w3782 w3786] -> w3600
              tunnel: [w3781 w3784] -> w3599
              tunnel: w3607 -> [w3781 w3787]
              tunnel: w3608 -> [w3782 w3788]
              frame False {
              }
              frame True {
                w3812 = i16 2 ("宽度(-)")
                w3813 = u32 100 ("y")
                w3807 = i16 2 ("宽度(-)")
                w3808 = u32 100 ("y")
                w3802 = u16 2 items=["byte", "word", "Dword"] ("数据类型")
                w3804 = u8 132 items=["I/O (P)"=128, "Input (I)"=129, "Output (Q)"=130, "Bit Memory (M)"=131, "Data (DB)"=132, "Instance Data (DI)"=133, "Local Data (L)"=134, "Predecessor Local Data (VL)"=135] ("寄存器类型")
                w3797 = u16 1 items=["byte", "word", "Dword"] ("数据类型")
                w3799 = u8 132 items=["I/O (P)"=128, "Input (I)"=129, "Output (Q)"=130, "Bit Memory (M)"=131, "Data (DB)"=132, "Instance Data (DI)"=133, "Local Data (L)"=134, "Predecessor Local Data (VL)"=135] ("寄存器类型")
                w3792 = u16 2 items=["byte", "word", "Dword"] ("数据类型")
                w3794 = u8 132 items=["I/O (P)"=128, "Input (I)"=129, "Output (Q)"=130, "Bit Memory (M)"=131, "Data (DB)"=132, "Instance Data (DI)"=133, "Local Data (L)"=134, "Predecessor Local Data (VL)"=135] ("寄存器类型")
                n2052 = call "S7_Read.vi"("TCP"=w3788, "DB #"=u16 20, "读取长度"=u16 9, "寄存器类型"=w3794, "起始地址"=u32 64, "数据类型"=w3792, "error in"=w3787) -> ("TCP"=w3814:refnum<k5>, "数据"=w3818:u32[], "error out"=w3815:errorcluster)  [unwired: 5 in, 1 out]
                n2053 = Index Array(array=w3818) -> (element #1=w3819:u32, element #2=w3827:u32, element #3=w3821:u32, element #4=w3822:u32, element #5=w3832:u32, element #6=w3833:u32, element #7=w3834:u32, element #8=w3836:u32, element #9=w3839:u32)  [unwired: 9 in]
                n2054 = Divide(x=w3833, y=w3808) -> (x/y=w3829:dbl)
                n2055 = Divide(x=w3832, y=w3808) -> (x/y=w3828:dbl)
                n2056 = Divide(x=w3827, y=w3808) -> (x/y=w3825:dbl)
                n2057 = Number To Decimal String(number=w3819) -> (decimal integer string=w3820:string)  [unwired: 1 in]
                n2058 = Number To Decimal String(number=w3821) -> (decimal integer string=w3823:string)  [unwired: 1 in]
                n2059 = Number To Decimal String(number=w3822) -> (decimal integer string=w3824:string)  [unwired: 1 in]
                n2060 = Number To Fractional String(number=w3825, precision (6)=w3807) -> (F-format string=w3826:string)  [unwired: 2 in]
                n2061 = Number To Fractional String(number=w3828, precision (6)=w3807) -> (F-format string=w3830:string)  [unwired: 2 in]
                n2062 = Number To Fractional String(number=w3829, precision (6)=w3807) -> (F-format string=w3831:string)  [unwired: 2 in]
                n2063 = Number To Decimal String(number=w3834) -> (decimal integer string=w3835:string)  [unwired: 1 in]
                n2064 = Number To Decimal String(number=w3836) -> (decimal integer string=w3837:string)  [unwired: 1 in]
                n2065 = Number To Decimal String(number=w3839) -> (decimal integer string=w3838:string)  [unwired: 1 in]
                n2066 = call "S7_Read.vi"("TCP"=w3814, "DB #"=u16 20, "读取长度"=u16 1, "寄存器类型"=w3799, "起始地址"=u32 100, "数据类型"=w3797, "error in"=w3815) -> ("TCP"=w3816:refnum<k5>, "数据"=w3840:u32[], "error out"=w3817:errorcluster)  [unwired: 5 in, 1 out]
                n2067 = Index Array(array=w3840) -> (element=w3842:u32)  [unwired: 1 in]
                n2068 = Equal?(x=w3842, y=u32 1) -> (x = y?=w3841:bool)
                n2069 = case shown="真" w3841 {
                  tunnel: ["NG" "OK"] -> w3845
                  frame False {
                  }
                  frame True {
                  }
                }
                n2070 = call "S7_Read.vi"("TCP"=w3816, "DB #"=u16 20, "读取长度"=u16 9, "寄存器类型"=w3804, "起始地址"=u32 102, "数据类型"=w3802, "error in"=w3817) -> ("TCP"=w3786:refnum<k5>, "数据"=w3858:u32[], "error out"=w3785:errorcluster)  [unwired: 5 in, 1 out]
                n2071 = Index Array(array=w3858) -> (element #1=w3857:u32, element #2=w3853:u32, element #3=w3856:u32, element #4=w3855:u32, element #5=w3850:u32, element #6=w3849:u32, element #7=w3848:u32, element #8=w3847:u32, element #9=w3846:u32)  [unwired: 9 in]
                n2072 = Divide(x=w3849, y=w3813) -> (x/y=w3851:dbl)
                n2073 = Divide(x=w3850, y=w3813) -> (x/y=w3852:dbl)
                n2074 = Divide(x=w3853, y=w3813) -> (x/y=w3854:dbl)
                n2075 = Format Date/Time String(time format string (%c)="%Y-%m-%d" ("时间格式字符串(%c)")) -> (date/time string=w3843:string)  [unwired: 2 in]
                n2076 = Get Date/Time String(want seconds? (F)=TRUE ("需要秒？(F)")) -> (time string=w3844:string)  [unwired: 2 in, 1 out]
                n2077 = Number To Decimal String(number=w3857) -> (decimal integer string=w3859:string)  [unwired: 1 in]
                n2078 = Number To Decimal String(number=w3856) -> (decimal integer string=w3860:string)  [unwired: 1 in]
                n2079 = Number To Decimal String(number=w3855) -> (decimal integer string=w3861:string)  [unwired: 1 in]
                n2080 = Number To Fractional String(number=w3854, precision (6)=w3812) -> (F-format string=w3862:string)  [unwired: 2 in]
                n2081 = Number To Fractional String(number=w3852, precision (6)=w3812) -> (F-format string=w3863:string)  [unwired: 2 in]
                n2082 = Number To Fractional String(number=w3851, precision (6)=w3812) -> (F-format string=w3864:string)  [unwired: 2 in]
                n2083 = Number To Decimal String(number=w3848) -> (decimal integer string=w3865:string)  [unwired: 1 in]
                n2084 = Number To Decimal String(number=w3847) -> (decimal integer string=w3866:string)  [unwired: 1 in]
                n2085 = Number To Decimal String(number=w3846) -> (decimal integer string=w3867:string)  [unwired: 1 in]
                n2086 = Insert Into Array(array=string[] [] ("数组"), index=0 ("索引"), new element #1="201" ("新元素/子数组"), new element #2=w3845, new element #3=w3843, new element #4=w3844, new element #5=w3845, new element #6=w3820, new element #7=w3823, new element #8=w3824, new element #9=w3826, new element #10=w3830, new element #11=w3831, new element #12=w3835, new element #13=w3837, new element #14=w3838, new element #15=w3859, new element #16=w3860, new element #17=w3861, new element #18=w3862, new element #19=w3863, new element #20=w3864, new element #21=w3865, new element #22=w3866, new element #23=w3867) -> (w3783:string[])
                n2087 = stacked-sequence {
                  tunnel: w3785 -> [_ w3873]
                  tunnel: [_ w3870] -> w3784
                  tunnel: w3783 -> [w3869 _]
                  frame #0 {
                    n2088 = local write "202数据回复写入"(FALSE ("202数据回复写入")) -> ()
                    "201数据" <- w3869
                  }
                  frame #1 {
                    n2089 = property on="ST201数据读取(事件)" class="Bool (严格)"(error in=w3873, "Val(Sgnl)"=TRUE ("值(信号)")) -> (error out=w3871:errorcluster)  [unwired: 1 in, 1 out]
                    n2090 = disable-structure shown="启用" {
                      disable-tunnel: w3871 -> [w3875 w3877]
                      disable-tunnel: [w3874 w3877] -> w3870
                      frame Disabled {
                        n2091 = property on="ST201画曲线" class="Bool (严格)"(error in=w3875, "Val(Sgnl)"=TRUE ("值(信号)")) -> (error out=w3874:errorcluster)  [unwired: 1 in, 1 out]
                      }
                      frame Enabled {
                      }
                    }
                  }
                }
              }
            }
            n2092 = call <vilib>:"Boolean Crossing PtByPt.vi"("direction"=enum16{"either", "false-true", "true-false"}."false-true", "input"=w3588) -> ("crossing"=w3598:bool)  [unwired: 1 in]
            n2093 = case shown="真" w3598 {
              tunnel: w3600 -> [w3759 w3764]
              tunnel: w3599 -> [w3758 w3763]
              tunnel: [w3758 w3762] -> w3596
              tunnel: [w3759 w3761] -> w3597
              frame False {
              }
              frame True {
                w3765 = u16 0 items=["byte", "word", "Dword"] ("数据类型")
                w3767 = u8 132 items=["I/O (P)"=128, "Input (I)"=129, "Output (Q)"=130, "Bit Memory (M)"=131, "Data (DB)"=132, "Instance Data (DI)"=133, "Local Data (L)"=134, "Predecessor Local Data (VL)"=135] ("寄存器类型")
                n2094 = call "S7_Read.vi"("TCP"=w3764, "DB #"=u16 20, "读取长度"=u16 13, "寄存器类型"=w3767, "起始地址"=u32 44, "数据类型"=w3765, "error in"=w3763) -> ("TCP"=w3761:refnum<k5>, "数据"=w3770:u32[], "error out"=w3772:errorcluster)  [unwired: 5 in, 1 out]
                n2095 = To Unsigned Word Integer(number=w3770) -> (unsigned 16bit integer=w3771:u16[])
                n2096 = call "还原为字符串.vi"("error in (no error)"=w3772, "输入数组"=w3771) -> ("error out"=w3773:errorcluster, "字符串"=w3760:string)  [unwired: 8 in]
                n2097 = stacked-sequence {
                  tunnel: w3773 -> [_ w3777]
                  tunnel: [_ w3775] -> w3762
                  tunnel: w3760 -> [w3774 _]
                  frame #0 {
                    "202二维码" <- w3774
                  }
                  frame #1 {
                    n2098 = property on="ST202扫码请求(事件)" class="Bool (严格)"(error in=w3777, "Val(Sgnl)"=TRUE ("值(信号)")) -> (error out=w3775:errorcluster)  [unwired: 1 in, 1 out]
                  }
                }
              }
            }
            n2099 = call <vilib>:"Boolean Crossing PtByPt.vi"("direction"=enum16{"either", "false-true", "true-false"}."false-true", "input"=w3587) -> ("crossing"=w3592:bool)  [unwired: 1 in]
            n2100 = case shown="真" w3592 {
              tunnel: w3597 -> [w3646 w3710]
              tunnel: w3596 -> [w3645 w3709]
              tunnel: [w3646 w3671] -> w3594
              tunnel: [w3645 w3648] -> w3595
              frame False {
              }
              frame True {
                w3654 = 15 ("长度")
                w3699 = u16 0 items=["byte", "word", "Dword"] ("数据类型")
                w3697 = u8 132 items=["I/O (P)"=128, "Input (I)"=129, "Output (Q)"=130, "Bit Memory (M)"=131, "Data (DB)"=132, "Instance Data (DI)"=133, "Local Data (L)"=134, "Predecessor Local Data (VL)"=135] ("寄存器类型")
                w3716 = u16 1 items=["byte", "word", "Dword"] ("数据类型")
                w3718 = u8 132 items=["I/O (P)"=128, "Input (I)"=129, "Output (Q)"=130, "Bit Memory (M)"=131, "Data (DB)"=132, "Instance Data (DI)"=133, "Local Data (L)"=134, "Predecessor Local Data (VL)"=135] ("寄存器类型")
                w3711 = u16 2 items=["byte", "word", "Dword"] ("数据类型")
                w3713 = u8 132 items=["I/O (P)"=128, "Input (I)"=129, "Output (Q)"=130, "Bit Memory (M)"=131, "Data (DB)"=132, "Instance Data (DI)"=133, "Local Data (L)"=134, "Predecessor Local Data (VL)"=135] ("寄存器类型")
                # "20的零件号"
                n2101 = call "S7_Read.vi"("TCP"=w3710, "DB #"=u16 20, "读取长度"=u16 6, "寄存器类型"=w3713, "起始地址"=u32 138, "数据类型"=w3711, "error in"=w3709) -> ("TCP"=w3730:refnum<k5>, "数据"=w3732:u32[], "error out"=w3731:errorcluster)  [unwired: 5 in, 1 out]
                n2102 = Index Array(array=w3732) -> (element #1=w3733:u32, element #2=w3708:u32, element #3=w3734:u32, element #4=w3735:u32, element #5=w3703:u32, element #6=w3701:u32)  [unwired: 6 in]
                n2103 = Divide(x=w3708, y=u32 100) -> (x/y=w3707:dbl)
                n2104 = Divide(x=w3703, y=u32 100) -> (x/y=w3702:dbl)
                n2105 = Divide(x=w3701, y=u32 100) -> (x/y=w3700:dbl)
                n2106 = Number To Decimal String(number=w3733) -> (decimal integer string=w3742:string)  [unwired: 1 in]
                n2107 = Number To Decimal String(number=w3734) -> (decimal integer string=w3743:string)  [unwired: 1 in]
                n2108 = Number To Decimal String(number=w3735) -> (decimal integer string=w3744:string)  [unwired: 1 in]
                n2109 = call "S7_Read.vi"("TCP"=w3730, "DB #"=u16 20, "读取长度"=u16 1, "寄存器类型"=w3718, "起始地址"=u32 162, "数据类型"=w3716, "error in"=w3731) -> ("TCP"=w3673:refnum<k5>, "数据"=w3736:u32[], "error out"=w3672:errorcluster)  [unwired: 5 in, 1 out]
                n2110 = Number To Fractional String(number=w3707, precision (6)=i16 2 ("精度(6)")) -> (F-format string=w3745:string)  [unwired: 2 in]
                n2111 = Number To Fractional String(number=w3702, precision (6)=i16 2 ("精度(6)")) -> (F-format string=w3746:string)  [unwired: 2 in]
                n2112 = Number To Fractional String(number=w3700, precision (6)=i16 2 ("精度(6)")) -> (F-format string=w3747:string)  [unwired: 2 in]
                n2113 = Index Array(array=w3736) -> (element=w3738:u32)  [unwired: 1 in]
                n2114 = Equal?(x=w3738, y=u32 1) -> (x = y?=w3737:bool)
                n2115 = case shown="真" w3737 {
                  tunnel: ["NG" "OK"] -> w3741
                  frame False {
                  }
                  frame True {
                  }
                }
                n2116 = Format Date/Time String(time format string (%c)="%Y-%m-%d" ("时间格式字符串(%c)")) -> (date/time string=w3739:string)  [unwired: 2 in]
                n2117 = Get Date/Time String(want seconds? (F)=TRUE ("需要秒？(F)")) -> (time string=w3740:string)  [unwired: 2 in, 1 out]
                n2118 = call "S7_Read.vi"("TCP"=w3673, "DB #"=u16 20, "读取长度"=u16 100, "寄存器类型"=w3697, "起始地址"=u32 164, "数据类型"=w3699, "error in"=w3672) -> ("TCP"=w3671:refnum<k5>, "数据"=w3655:u32[], "error out"=w3670:errorcluster)  [unwired: 5 in, 1 out]
                n2119 = Delete From Array(array=w3655, length=w3654, index=2 ("索引")) -> (deleted portion=w3676:u32[])  [unwired: 1 out]
                n2120 = Delete From Array(array=w3655, length=w3654, index=22 ("索引")) -> (deleted portion=w3675:u32[])  [unwired: 1 out]
                n2121 = Delete From Array(array=w3655, length=w3654, index=42 ("索引")) -> (deleted portion=w3674:u32[])  [unwired: 1 out]
                n2122 = Delete From Array(array=w3655, length=w3654, index=82 ("索引")) -> (deleted portion=w3656:u32[])  [unwired: 1 out]
